vi "Ramp Generator.vi"(4 "Channel Data":T3(array[cluster]) {"Gauge Length" format="%.2f"; "Full Scale" format="%.2f"; "SI Full Scale" format="%.2f"}, 7 "Input cluster":T1 {"Set Point" format="%.2f"; "Ramp Amplitude" format="%.2f"; "Ramp Rate" format="%.2f"; "Set Point Time" format="%.2f"}, 8 "error in (no error)":errorcluster, 9 "Channels":u16[](array[ring]) items=["Channel 1", "Channel 2", "Channel 3", "Channel 4"], 10 "Axis Selector":i32[](listbox), 11 "Axis Information":T2(array[cluster])) -> (0 "Error Out":errorcluster, 1 "Channels Out":u16[](array[ring]) items=["Channel 1", "Channel 2", "Channel 3", "Channel 4"], 2 "Axis Selector Out":i32[](listbox), 3 "Axis Information Out":T2(array[cluster]))   [LabVIEW 2011]
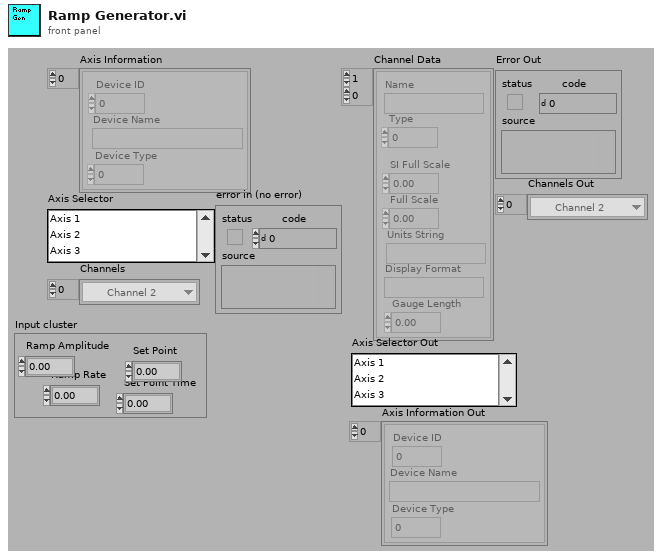
[diagram p1: front panel]
types:
  T1 = cluster{"Set Point":dbl, "Set Point Time":dbl, "Ramp Amplitude":dbl, "Ramp Rate":dbl}
  T2 = cluster{"Device ID":i32, "Device Name":string, "Device Type":i32}[]
  T3 = cluster{"Name":string, "Type":i32, "SI Full Scale":dbl, "Full Scale":dbl, "Units String":string, "Display Format":string, "Gauge Length":dbl}[][]
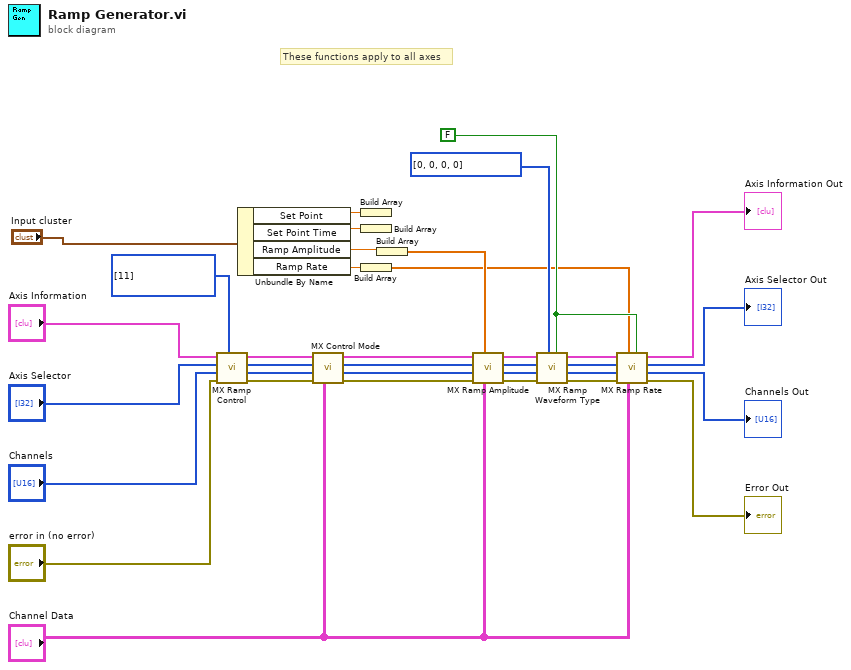
[diagram p0: block diagram]
diagram:
  w1 = u16[] [11] items=["Stop", "Start or continue", "Hold", "Continue", "Return ramp to set level at fixed rate", "Reserved", "Reserved", "Start Random without demand hold", "Start Random with demand hold", "Prepare Random Start without demand hold", "Prepare Random Start with demand hold", "Unslave", "Reserved", "Reserved", "Start Sample Data Playback or Resume", "Prepare for Start of Sample Data", "Reserved", "Reserved", "Resume Playback", "Start an electromechanical frame return"] ("Ramp Control")
  w22 = FALSE ("Next?")
  w27 = u16[] [0, 0, 0, 0] items=["Ramp", "Dual Ramp", "Trapezium", "Absolute Ramp", "Hold Ramp", "Absolute Rate Ramp"] ("Waveform Types")
  # "These functions apply to all axes"
  n1 = call "MX Ramp Control.vi"("Ramp Control"=w1, "error in (no error)"="error in (no error)", "Channels In"="Channels", "Axis Selector In"="Axis Selector", "Axis Information In"="Axis Information") -> ("error out"=w32:errorcluster, "Channels Out"=w33:u16[], "Axis Selector Out"=w34:i32[], "Axis Information Out"=w35:T2)  [unwired: 2 in]
  n2 = Unbundle By Name("Input cluster") -> ("Set Point"=w12:dbl, "Set Point Time"=w11:dbl, "Ramp Amplitude"=w10:dbl, "Ramp Rate"=w8:dbl)
  n3 = call "MX Control Mode.vi"("Channel Data"="Channel Data", "error in (no error)"=w32, "Control Modes"=w33, "Axis Selector"=w34, "Axis Information"=w35) -> ("error out"=w2:errorcluster, "Control Modes out"=w3:u16[], "Axis Selector out"=w4:i32[], "Axis Information out"=w5:T2)  [unwired: 1 in]
  n4 = Build Array(w12) -> ()  [unwired: 1 out]
  n5 = Build Array(w11) -> ()  [unwired: 1 out]
  n6 = Build Array(w8) -> (w7:dbl[])
  n7 = Build Array(w10) -> (w9:dbl[])
  n8 = call "MX Ramp Amplitude.vi"("Channel Data"="Channel Data", "Ramp Amplitude"=w9, "error in (no error)"=w2, "Channels In"=w3, "Axis Selector In"=w4, "Axis Information In"=w5) -> ("error out"=w29:errorcluster, "Channels Out"=w30:u16[], "Axis Selector Out"=w31:i32[], "Axis Information Out"=w28:T2)  [unwired: 1 in]
  n9 = call "MX Ramp Waveform Type.vi"("Next?"=w22, "Waveform Types"=w27, "error in (no error)"=w29, "Channels In"=w30, "Axis Selector In"=w31, "Axis Information In"=w28) -> ("error out"=w23:errorcluster, "Channels Out"=w24:u16[], "Axis Selector Out"=w25:i32[], "Axis Information Out"=w26:T2)  [unwired: 1 in]
  n10 = call "MX Ramp Rate.vi"("Next?"=w22, "Channel Data"="Channel Data", "Ramp Rate"=w7, "error in (no error)"=w23, "Channels In"=w24, "Axis Selector In"=w25, "Axis Information In"=w26) -> ("error out"=→"Error Out":errorcluster, "Channels Out"=→"Channels Out":u16[], "Axis Selector Out"=→"Axis Selector Out":i32[], "Axis Information Out"=→"Axis Information Out":T2)
